vi "New.vi"(8 "error in (no error)":errorcluster, 11 "reference in":refnum<class "TestCSMSuite.lvclass">) -> (0 "error out":errorcluster, 3 "reference out":refnum<class "TestCSMSuite.lvclass">)   [LabVIEW 2017, in "TestCSMSuite.lvclass"]
uses:
  TestCSMSuite.lvclass
  C:/Program Files (x86)/National Instruments/LabVIEW 2017/vi.lib/addons/_JKI Toolkits/VI Tester/TestSuite.llb/TestSuite.lvclass
  <vilib>/addons/_JKI Toolkits/VI Tester/TestCase.llb/TestCase.lvclass
  testcase-CSMManagementAPI/testcase-CSMManagementAPI.lvclass
  C:/Program Files (x86)/National Instruments/LabVIEW 2017/vi.lib/addons/_JKI Toolkits/VI Tester/TestCase.llb/TestCase.lvclass
  testcase-CSMArgument/testcase-CSMArgument.lvclass
  testcase-CSMMessage/testcase-CSMMessage.lvclass
  testcase-CSMResponse/testcase-CSMResponse.lvclass
  testcase-CSMSubModule/testcase-CSMSubModule.lvclass
  testcase-CSMWorkerMode/testcase-CSMWorkerMode.lvclass
  testcase-CSMChainMode/testcase-CSMChainMode.lvclass
  testcase-CSMNonCSMCallerSupportAPI/testcase-CSMNonCSMCallerSupportAPI.lvclass
  testcase-CSMAddonLoopSupport/testcase-CSMAddonLoopSupport.lvclass
  testcase-CSMGlobalLog/testcase-CSMGlobalLog.lvclass
  testcase-CSMSystemLevelModule/testcase-CSMSystemLevelModule.lvclass
  testcase-CSMBroadcast/testcase-CSMBroadcast.lvclass
  TestCSMSuite.lvclass/TestCSMSuite.ctl
  <vilib>/addons/_JKI Toolkits/VI Tester/TestSuite.llb/TestSuite.lvclass
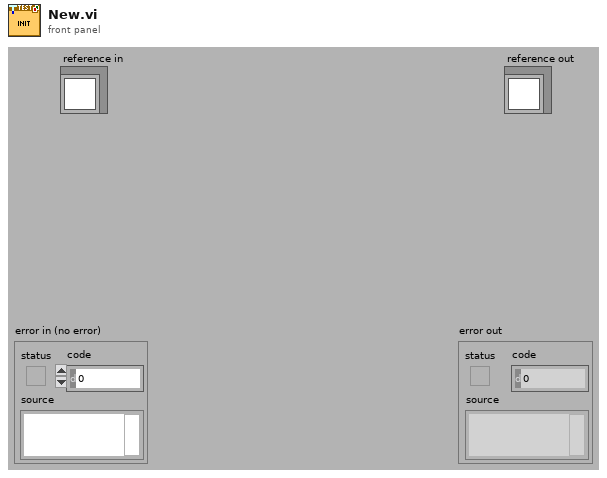
[diagram p1: front panel]
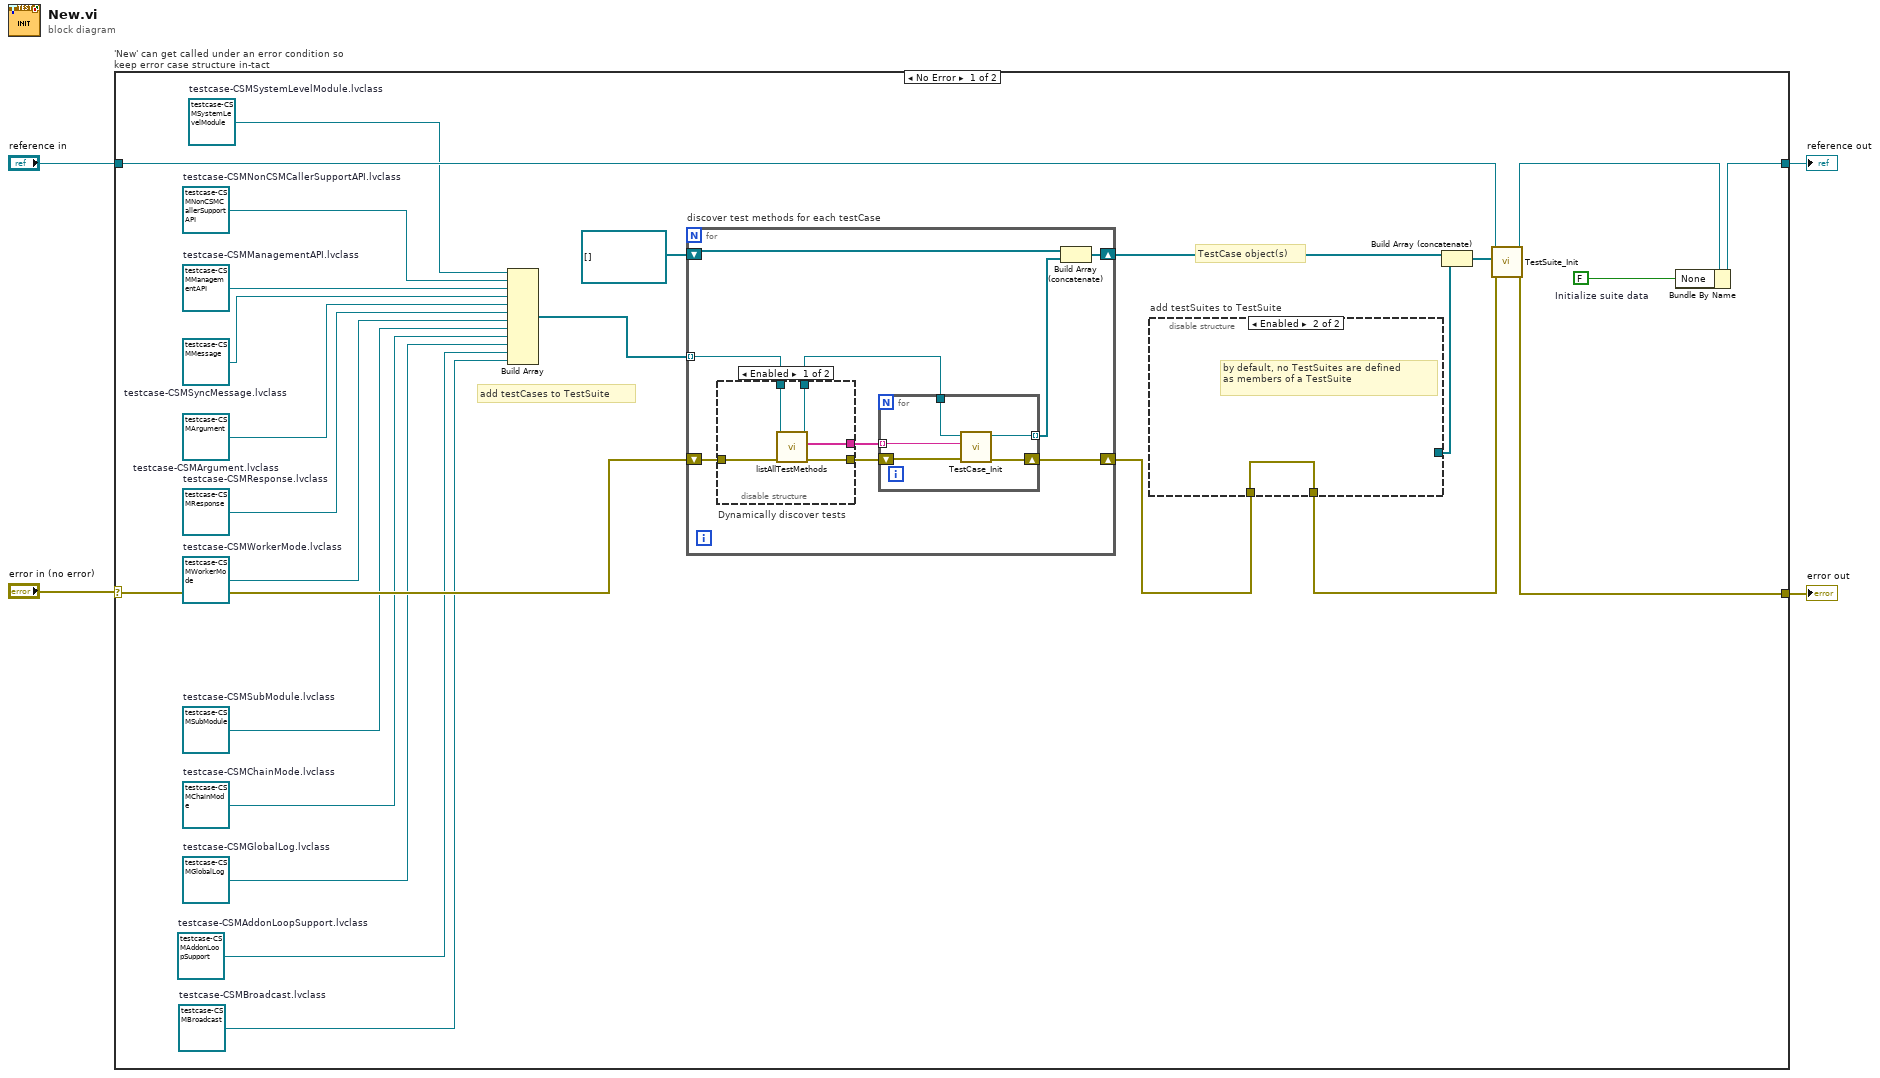
[diagram p0: block diagram]
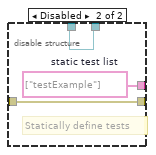
[diagram p2: hidden frame]
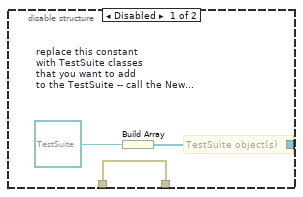
[diagram p3: hidden frame]
diagram:
  n1 = case "'New' can get called under an error condition so keep error case structure in-tact" shown="No Error" "error in (no error)" {
    selector: "error in (no error)" -> [w23 w56]
    tunnel: [w29 w57] -> w4
    tunnel: "reference in" -> [w24 w57]
    tunnel: [w26 w56] -> w1
    frame No Error {
      w5 = refnum<class "testcase-CSMBroadcast.lvclass"> refnum  # testcase-CSMBroadcast.lvclass
      w7 = refnum<class "testcase-CSMSystemLevelModule.lvclass"> refnum  # testcase-CSMSystemLevelModule.lvclass
      w9 = refnum<class "testcase-CSMGlobalLog.lvclass"> refnum  # testcase-CSMGlobalLog.lvclass
      w6 = refnum<class "testcase-CSMAddonLoopSupport.lvclass"> refnum  # testcase-CSMAddonLoopSupport.lvclass
      w8 = refnum<class "testcase-CSMNonCSMCallerSupportAPI.lvclass"> refnum  # testcase-CSMNonCSMCallerSupportAPI.lvclass
      w10 = refnum<class "testcase-CSMChainMode.lvclass"> refnum  # testcase-CSMChainMode.lvclass
      w12 = refnum<class "testcase-CSMWorkerMode.lvclass"> refnum  # testcase-CSMWorkerMode.lvclass
      w11 = refnum<class "testcase-CSMSubModule.lvclass"> refnum  # testcase-CSMSubModule.lvclass
      w13 = refnum<class "testcase-CSMResponse.lvclass"> refnum  # testcase-CSMResponse.lvclass
      w15 = refnum<class "testcase-CSMMessage.lvclass"> refnum  # testcase-CSMSyncMessage.lvclass
      w14 = refnum<class "testcase-CSMArgument.lvclass"> refnum  # testcase-CSMArgument.lvclass
      w16 = refnum<class "testcase-CSMManagementAPI.lvclass"> refnum  # testcase-CSMManagementAPI.lvclass
      w28 = FALSE  # Initialize suite data
      # "TestCase object(s)"
      # "add testCases to TestSuite"
      n2 = Build Array(w7, w8, w16, w15, w14, w13, w12, w11, w10, w9, w6, w5) -> (w25:refnum<class "TestCase.lvclass">[])
      n3 = for "discover test methods for each testCase" {
        shift-right: [w38] -> w18
        shift-left: w23 -> [w34]
        tunnel: w25 -> [w31] mode=indexing
        shift-right: [w35] -> w22
        shift-left: refnum<class "TestCase.lvclass">[] [] -> [w36]
        n4 = disable-structure "Dynamically discover tests" shown="Enabled" {
          disable-tunnel: w34 -> [w43 w44]
          disable-tunnel: [w42 w44] -> w33
          disable-tunnel: [w41 w45] -> w32
          disable-tunnel: w31 -> [w40 w46]
          disable-tunnel: [w39 w46] -> w30
          frame Enabled {
            n5 = call-dynamic "listAllTestMethods.vi"("error in (no error)"=w43, "TestCase in"=w40) -> ("error out"=w42:errorcluster, "test methods"=w41:string[], "TestCase out"=w39:refnum<class "TestCase.lvclass">)  [unwired: 7 in]
          }
          frame Disabled {
            w45 = string[] ["testExample"]  # static test list
            # "Statically define tests"
          }
        }
        n6 = for {
          tunnel: w30 -> [w47]
          tunnel: w32 -> [w51] mode=indexing
          shift-right: [w49] -> w38
          shift-left: w33 -> [w50]
          tunnel: [w48] -> w37 mode=indexing
          n7 = call <vilib>:"TestCase_Init.vi"("error in (no error)"=w50, "methodName (\"runTest\")"=w51, "TestCase in"=w47) -> ("error out"=w49:errorcluster, "TestCase out"=w48:refnum<class "TestCase.lvclass">)  [unwired: 7 in]
        }
        n8 = Build Array (concatenate)(w36, w37) -> (w35:refnum<class "TestCase.lvclass">[])
      }
      n9 = disable-structure "add testSuites to TestSuite" shown="Enabled" {
        disable-tunnel: [w52 _] -> w20
        disable-tunnel: [w54 w55] -> w19
        disable-tunnel: w18 -> [w54 w55]
        frame Disabled {
          w53 = refnum<class "TestSuite.lvclass"> refnum  # replace this constant with TestSuite classes that you want to add to the TestSuite -- call the New method for each TestSuite prior to adding it to this TestSuite
          # "TestSuite object(s)"
          n10 = Build Array(w53) -> (w52:refnum<class "TestSuite.lvclass">[])
        }
        frame Enabled {
          # "by default, no TestSuites are defined\nas members of a TestSuite"
        }
      }
      n11 = Build Array (concatenate)(w22, w20) -> (w21:refnum<class>[])
      n12 = call <vilib>:"TestSuite_Init.vi"("error in (no error)"=w19, "tests (none)"=w21, "TestSuite in"=w24) -> ("error out"=w26:errorcluster, "TestSuite out"=w27:refnum<class "TestCSMSuite.lvclass">)  [unwired: 7 in]
      n13 = Bundle By Name(cluster=w27, "None"=w28) -> (w29:refnum<class "TestCSMSuite.lvclass">)
    }
    frame Error {
    }
  }
  "reference out" <- w4
  "error out" <- w1
